vi "Configure Clock Recovery (Constant Frequency).vi"(7 "Enable Clock Recovery (T: Enable)":bool=TRUE, 8 "error in (no error)":errorcluster, 9 "Data Rate (2.5E+9)":dbl=2500000000.0, 10 "Clock Recovery Method (0: Fully Automatic)":i32(ring) items=["Fully Automatic", "Semi Automatic", "Manual"], 11 "VISA resource name":refnum<visa-resource-name>) -> (0 "error out":errorcluster, 3 "VISA resource name out":refnum<visa-resource-name>)   [LabVIEW 2016, in "Agilent 2000 3000 X-Series.lvlib"]
doc: "Configures clock recovery assuming the clock to be a constant frequency.\n\n<b>Note:</b>\nThis VI is specific to the 6000-X Series oscilloscopes. These features are not available on other models. Use <b>Configure Math Function Characteristics</b> and <b>Configure Math Function Source</b> before running this vi to set <b>Clock Recovery</b> as the math function and select the desired source."
uses:
  Agilent 2000 3000 X-Series.lvlib
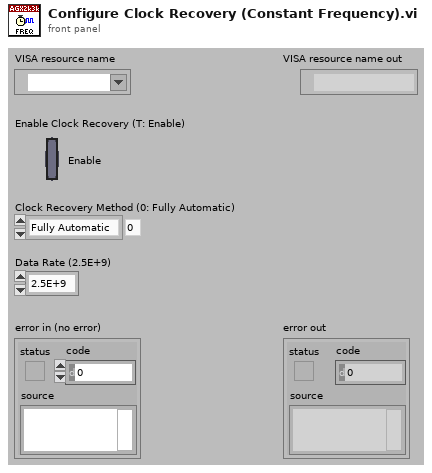
[diagram p1: front panel]
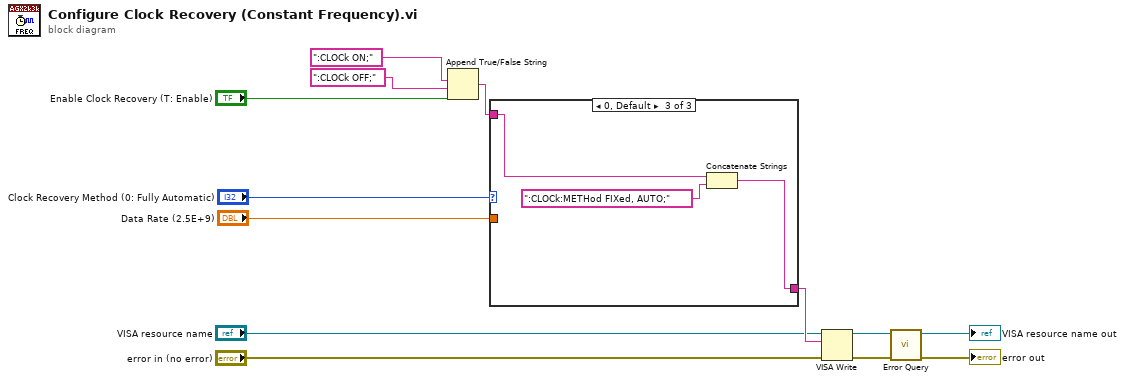
[diagram p0: block diagram]
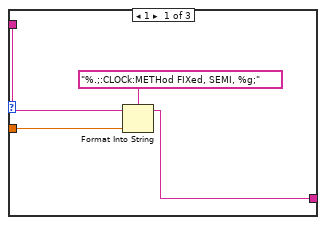
[diagram p2: hidden frame]
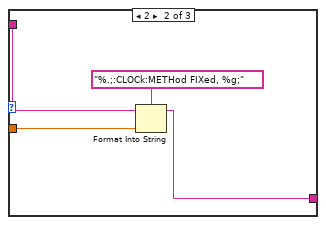
[diagram p3: hidden frame]
diagram:
  n1 = Append True/False String(1:"Enable Clock Recovery (T: Enable)", 2:":CLOCk OFF;", 3:":CLOCk ON;") -> (0:w10:string)  [unwired: 1 in]
  n2 = case shown="0, Default" "Clock Recovery Method (0: Fully Automatic)" {
    tunnel: w10 -> [w17 w21 w24]
    tunnel: "Data Rate (2.5E+9)" -> [w14 w18 _]
    tunnel: [w15 w19 w22] -> w8
    frame 1 {
      n3 = Format Into String(format string="%.;:CLOCk:METHod FIXed, SEMI, %g;", initial string=w17, w14) -> (resulting string=w15:string)  [unwired: 1 in, 1 out]
    }
    frame 2 {
      n4 = Format Into String(format string="%.;:CLOCk:METHod FIXed, %g;", initial string=w21, w18) -> (resulting string=w19:string)  [unwired: 1 in, 1 out]
    }
    frame 0, Default {
      n5 = Concatenate Strings(w24, ":CLOCk:METHod FIXed, AUTO;") -> (w22:string)
    }
  }
  n6 = VISA Write(VISA resource name="VISA resource name", write buffer=w8, error in (no error)="error in (no error)") -> (VISA resource name out=w4:refnum<visa-resource-name>, error out=w3:errorcluster)  [unwired: 1 out]
  n7 = call "Error Query.vi"("error in (no error)"=w3, "VISA resource name"=w4) -> ("error out"=→"error out":errorcluster, "VISA resource name out"=→"VISA resource name out":refnum<visa-resource-name>)  [unwired: 6 in, 2 out]
